vi "WFM - XSCAN.vi"(5 "Sampling Rate":dbl, 7 "Fast axis frequency":dbl=100.0, 8 "error in (no error)":errorcluster, 10 "Special coordinates (um)":T1, 11 "Frame Properties":T2={"Height (um)"=50.0, "Width (um)"=50.0, "Y Position (um)"=0.0, "X Position (um)"=0.0, "Y Resolution"=512.0}) -> (0 "error out":errorcluster, 2 "number of samples":dbl, 3 "signal out":waveform(dbl))   [LabVIEW 2017]
uses:
  <vilib>/measure/NI_MABase.lvlib
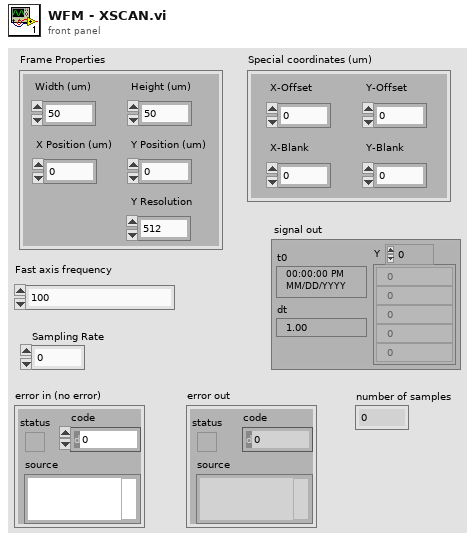
[diagram p1: front panel]
types:
  T1 = cluster{"Y-Offset":dbl, "X-Offset":dbl, "Y-Blank":dbl, "X-Blank":dbl}
  T2 = cluster{"Height (um)":dbl, "Width (um)":dbl, "Y Position (um)":dbl, "X Position (um)":dbl, "Y Resolution":dbl}
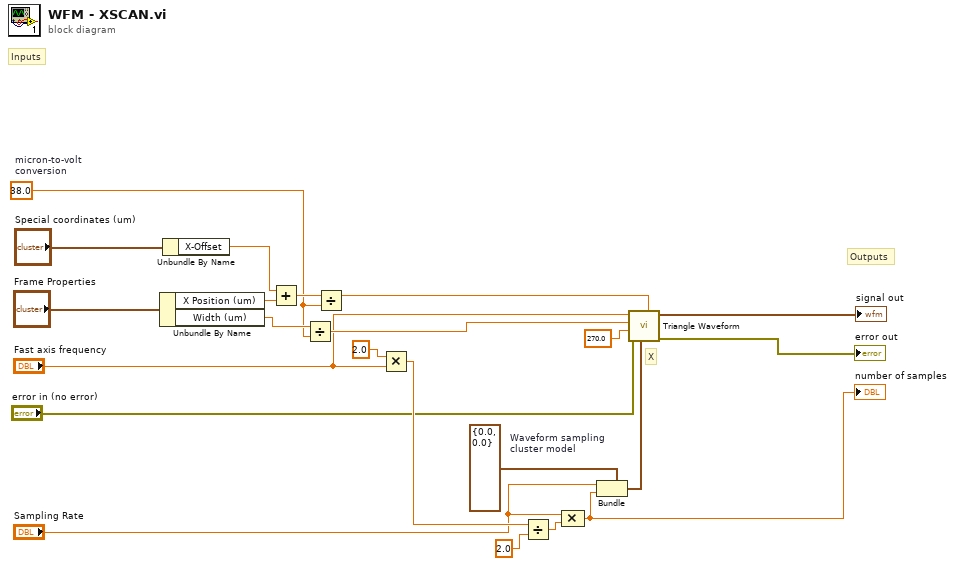
[diagram p0: block diagram]
diagram:
  w5 = 38.0  # micron-to-volt  conversion
  w14 = cluster{"Fs":dbl, "#s":dbl} {"Fs"=0.0, "#s"=0.0}  # Waveform sampling  cluster model
  # "Inputs"
  # "Outputs"
  # "X"
  n1 = Unbundle By Name("Frame Properties") -> ("X Position (um)"=w8:dbl, "Width (um)"=w22:dbl)
  n2 = Unbundle By Name("Special coordinates (um)") -> ("X-Offset"=w9:dbl)
  n3 = Add(x=w9, y=w8) -> (x+y=w6:dbl)
  n4 = Divide(x=w22, y=w5) -> (x/y=w21:dbl)
  n5 = Divide(x=w6, y=w5) -> (x/y=w7:dbl)
  n6 = Multiply(x=2.0 ("y"), y="Fast axis frequency") -> (x*y=w12:dbl)
  n7 = Divide(x=w12, y=2.0) -> (x/y=w15:dbl)
  n8 = Compound Arithmetic op=MULTIPLY("Sampling Rate", w15) -> (w17:dbl)
  "number of samples" <- w17
  n9 = Bundle(cluster=w14, "Fs"="Sampling Rate", "#s"=w17) -> (w13:cluster{"Fs":dbl, "#s":dbl})
  n10 = call <vilib>:"Triangle Waveform.vi"("offset"=w7, "sampling info"=w13, "error in (no error)"="error in (no error)", "phase"=270.0, "amplitude"=w21, "frequency"="Fast axis frequency") -> ("error out"=→"error out":errorcluster, "signal out"=→"signal out":waveform(dbl))  [unwired: 4 in]
